vi "ResMgr-RequestDef.vi"() -> (0 "ResMgr-RequestDef.ctl":T1)   [LabVIEW 2017, in "Communicable State Machine.lvlib"]
uses:
  Communicable State Machine.lvlib
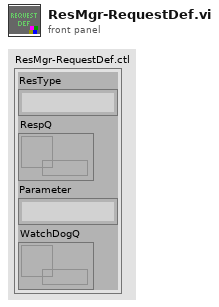
[diagram p1: front panel]
types:
  T1 = cluster{"ResType":string, "RespQ":refnum<queue>, "Parameter":string, "WatchDogQ":refnum<queue>}
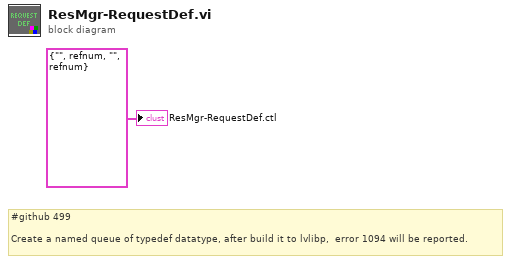
[diagram p0: block diagram]
diagram:
  # "#github 499\n\nCreate a named queue of typedef datatype, after build it to lvlibp,  error 1094 will be reported."
  "ResMgr-RequestDef.ctl" <- T1 {"ResType"="", "RespQ"=refnum, "Parameter"="", "WatchDogQ"=refnum} ("ResMgr-RequestDef.ctl")
